vi "Process_SpectralEmissionGateSweep.vi"(3 "Center WL":dbl format="%#_13g", 5 "Gate Start":dbl, 7 "Gate Width":dbl, 9 "Image":dbl[][][](array[numeric]), 13 "ColumnCalibration":dbl[](array[numeric]), 14 "WL width":dbl format="%#_13g") -> (6 "Gate Delay Array":dbl[](array[numeric]), 8 "Integrated emission vs gate delay":dbl[](array[numeric]), 15 "Spectra Array":dbl[][](array[numeric]))   [LabVIEW 2018]
uses:
  <vilib>/Analysis/baseanly.llb/Mean (DBL).vi
  <vilib>/Analysis/NI_AALBase.lvlib
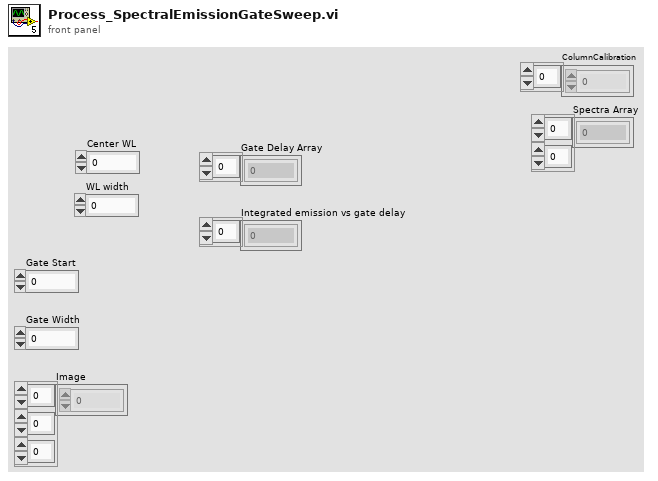
[diagram p1: front panel]
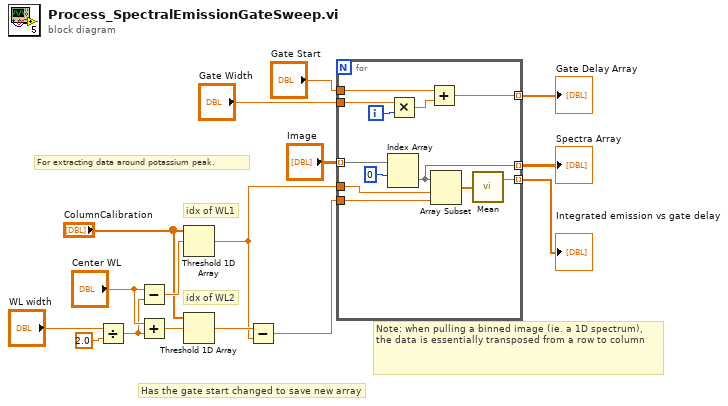
[diagram p0: block diagram]
diagram:
  # "idx of WL2"
  # "idx of WL1"
  # "For extracting data around potassium peak."
  # "Has the gate start changed to save new array"
  # "Note: when pulling a binned image (ie. a 1D spectrum), the data is essentially transposed from a row to column"
  n1 = Divide(x="WL width", y=2.0) -> (x/y=w8:dbl)
  n2 = Subtract(x="Center WL", y=w8) -> (x-y=w7:dbl)
  n3 = Add(x="Center WL", y=w8) -> (x+y=w6:dbl)
  n4 = Threshold 1D Array(2:w7, 3:"ColumnCalibration") -> (0:w3:dbl)  [unwired: 1 in]
  n5 = Threshold 1D Array(2:w6, 3:"ColumnCalibration") -> (0:w4:dbl)  [unwired: 1 in]
  n6 = Subtract(x=w4, y=w3) -> (x-y=w2:dbl)
  n7 = for {
    tunnel: "Image" -> [w22] mode=indexing
    tunnel: [w28] -> w13 mode=indexing
    tunnel: "Gate Start" -> [w24]
    tunnel: "Gate Width" -> [w26]
    tunnel: [w23] -> w14 mode=indexing
    tunnel: w3 -> [w20]
    tunnel: w2 -> [w19]
    tunnel: [w17] -> w1 mode=indexing
    i -> [w27]
    n8 = Index Array(array=w22, index (row)=0) -> (element=w17:dbl[])  [unwired: 1 in]
    n9 = Multiply(x=w26, y=w27) -> (x*y=w25:dbl)
    n10 = Add(x=w24, y=w25) -> (x+y=w23:dbl)
    n11 = Array Subset(array=w17, index=w20, length=w19) -> (w18:dbl[])
    n12 = call-poly <vilib>:"Mean.vi"("X"=w18) -> ("mean"=w28:dbl)  [unwired: 1 out]
  }
  "Gate Delay Array" <- w14
  "Integrated emission vs gate delay" <- w13
  "Spectra Array" <- w1
